vi "Create Shared Variable (Network).vi"(8 "error in (no error)":errorcluster, 9 "data type":T1(ring)=enum."double", 10 "shared variable name":string, 11 "process name":string) -> (0 "error out":errorcluster, 2 "variable reference out":refnum<k21>, 3 "process name out":string)   [LabVIEW 2018, in "Dynamic Shared Variables.lvlib"]
uses:
  Dynamic Shared Variables.lvlib
  <vilib>/lvdsc/NI_DSC.lvlib
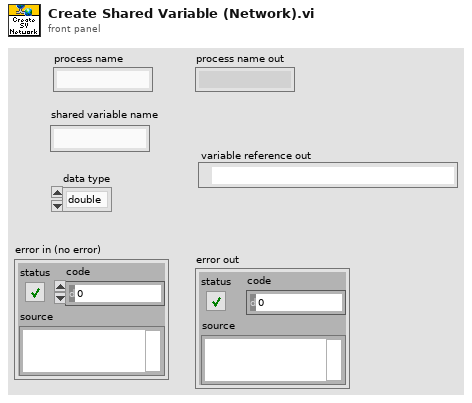
[diagram p1: front panel]
types:
  T1 = enum32{"u32BitField", "bool", "double", "string", "int8", "uint8", "int16", "uint16", "int32", "uint32", "int64", "uint64", "single", "double waveform", "int16 waveform", "array of boolean", "array of int8", "array of uint8", "array of int16", "array of uint16", "array of int32", "array of uint32", "array of int64", "array of uint64", "array of single", "array of double", "array of double waveform", "array of int16 waveform", "array of string", "variant", "timestamp", "fixed point", "custom"}
  T2 = cluster{"use binding? (F)":bool, "URL":string, "access type":enum32{"Read only", "Write only", "Read/write"}, "buffer size":u32, "use buffering? (F)":bool, "single writer? (F)":bool}
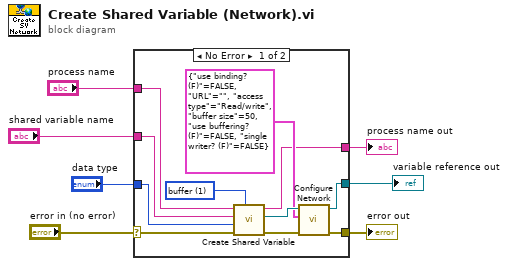
[diagram p0: block diagram]
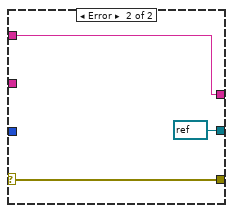
[diagram p2: hidden frame]
diagram:
  n1 = case shown="No Error" "error in (no error)" {
    selector: "error in (no error)" -> [w11 w20]
    tunnel: [w12 w21] -> w7
    tunnel: [w14 w20] -> w6
    tunnel: "process name" -> [w13 w21]
    tunnel: "shared variable name" -> [w10 _]
    tunnel: "data type" -> [w9 _]
    tunnel: [w8 refnum<k21> refnum ("variable reference out")] -> w1
    frame No Error {
      w18 = u16 1 items=["commit", "buffer"] ("set mode")
      n2 = call <vilib>:"Create Shared Variable.vi"("set mode"=w18, "error in (no error)"=w11, "data type"=w9, "shared variable name"=w10, "process name"=w13) -> ("error out"=w16:errorcluster, "shared variable"=w17:refnum<k21>, "process name out"=w12:string)  [unwired: 4 in]
      n3 = call <vilib>:"Configure Network.vi"("error in (no error)"=w16, "network settings"=T2 {"use binding? (F)"=FALSE, "URL"="", "access type"=enum."Read/write", "buffer size"=50, "use buffering? (F)"=FALSE, "single writer? (F)"=FALSE}, "variable reference in"=w17) -> ("error out"=w14:errorcluster, "variable reference out"=w8:refnum<k21>)  [unwired: 7 in]
    }
    frame Error {
    }
  }
  "process name out" <- w7
  "error out" <- w6
  "variable reference out" <- w1
